vi "bf.vi"() -> ()   [LabVIEW 2012]
panel:
  in  "Standard Input":string
  out "Standard Output":string
  in  "Source Code":string
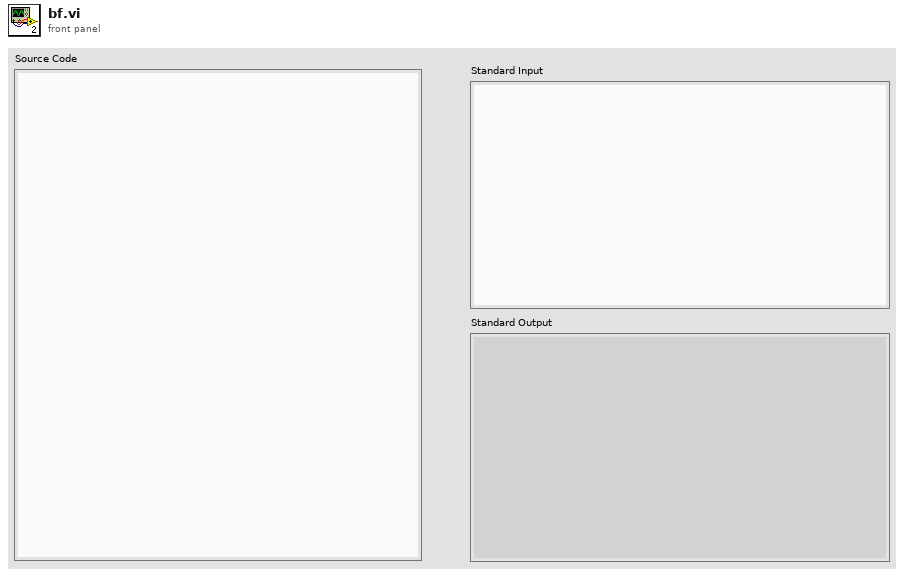
[diagram p1: front panel]
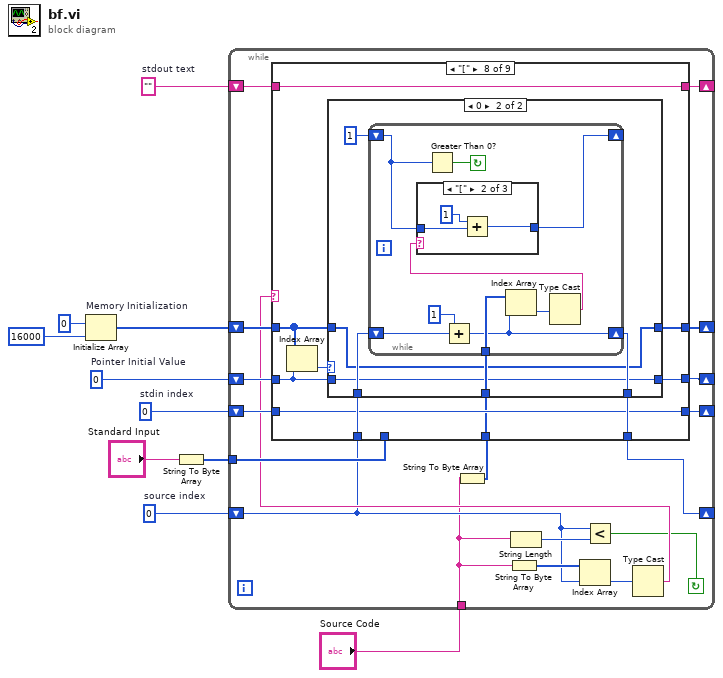
[diagram p0: block diagram]
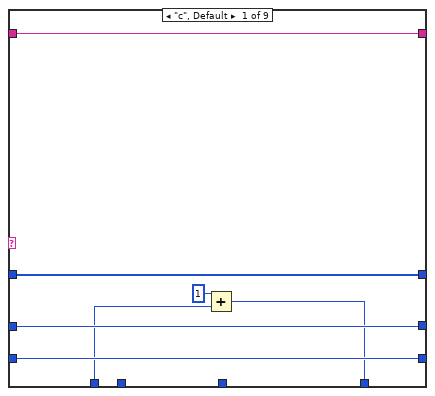
[diagram p2: hidden frame]
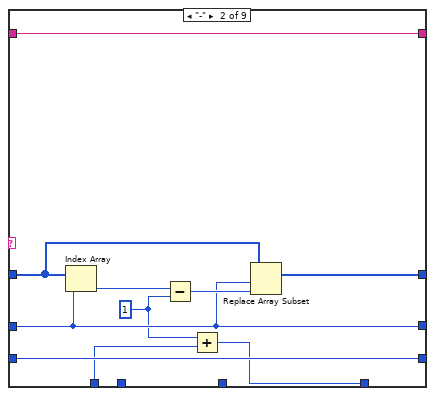
[diagram p3: hidden frame]
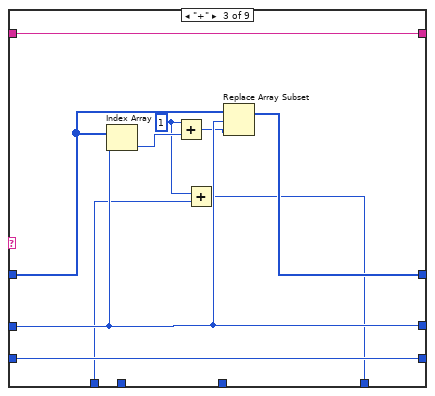
[diagram p4: hidden frame]
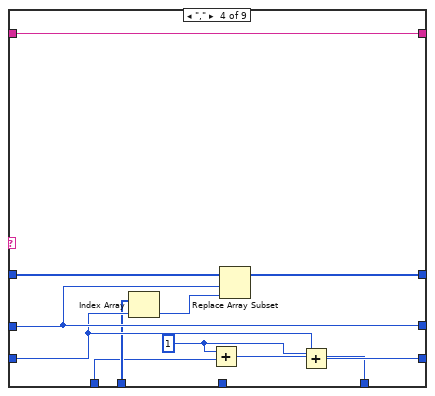
[diagram p5: hidden frame]
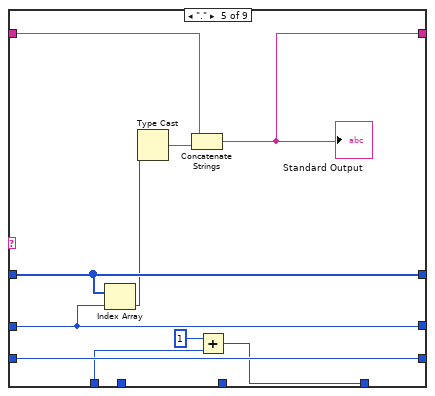
[diagram p6: hidden frame]
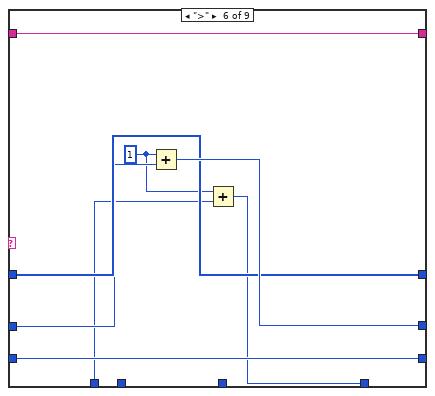
[diagram p7: hidden frame]
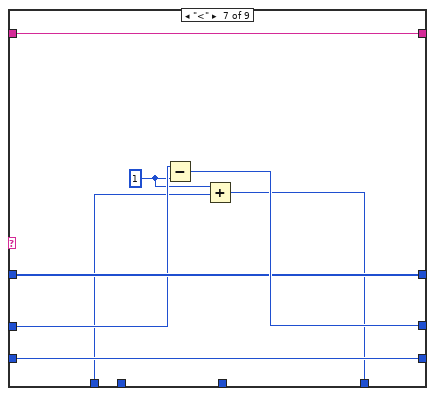
[diagram p8: hidden frame]
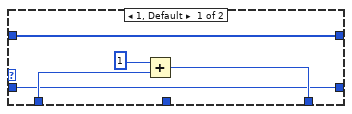
[diagram p9: hidden frame]
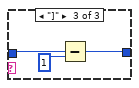
[diagram p11: hidden frame]
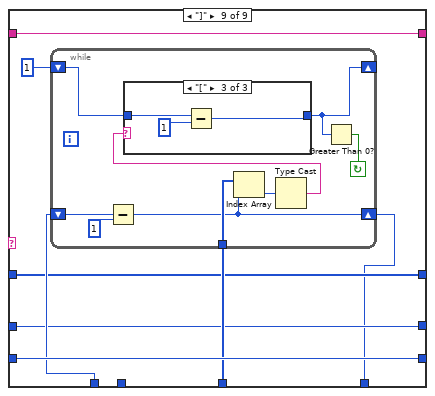
[diagram p12: hidden frame]
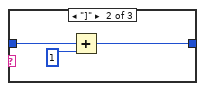
[diagram p14: hidden frame]
diagram:
  w1 = 0  # source index
  w4 = ""  # stdout text
  w5 = 0  # stdin index
  w8 = 0  # Pointer Initial Value
  n1 = Initialize Array "Memory Initialization"(u16 0, 16000) -> (w9:u16[])
  n2 = String To Byte Array(string="Standard Input") -> (unsigned byte array=w6:u8[])
  n3 = while {
    tunnel: "Source Code" -> [w12]
    shift-right: [w28] -> _
    shift-left: w8 -> [w25]
    shift-right: [w26] -> _
    shift-left: w9 -> [w27]
    tunnel: w6 -> [w22]
    shift-right: [w23] -> _
    shift-left: w5 -> [w24]
    shift-right: [w21] -> _
    shift-left: w4 -> [w20]
    shift-right: [w19] -> _
    shift-left: w1 -> [w13]
    stop <- w15 continue-if-true
    n4 = String To Byte Array(string=w12) -> (unsigned byte array=w11:u8[])
    n5 = String To Byte Array(string=w12) -> (unsigned byte array=w18:u8[])
    n6 = String Length(string=w12) -> (length=w14:i32)
    n7 = Index Array(array=w18, index=w13) -> (element=w16:u8)
    n8 = Less?(x=w13, y=w14) -> (x < y?=w15:bool)
    n9 = Type Cast(x=w16) -> (*(type *) &x=w17:string)  [unwired: 1 in]
    n10 = case shown="\"[\"" w17 {
      tunnel: [w34 w41 w52 w64 w75 w84 w92 w93 w131] -> w28
      tunnel: w27 -> [w35 w45 w53 w66 w76 w83 w91 w96 w132]
      tunnel: [w35 w44 w54 w65 w76 w83 w91 w95 w132] -> w26
      tunnel: w25 -> [w34 w41 w52 w64 w75 w82 w89 w94 w131]
      tunnel: w24 -> [w33 w40 w50 w63 w73 w81 w90 w99 w135]
      tunnel: [w33 w40 w50 w62 w73 w81 w90 w99 w135] -> w23
      tunnel: w22 -> [_ _ _ w61 _ _ _ _ _]
      tunnel: [w32 w39 w49 w59 w70 w80 w88 w97 w137] -> w21
      tunnel: w20 -> [w32 w39 w49 w59 w72 w80 w88 w97 w137]
      tunnel: w13 -> [w30 w37 w46 w57 w68 w78 w86 w101 w134]
      tunnel: [w29 w36 w47 w58 w69 w77 w85 w100 w130] -> w19
      tunnel: w11 -> [_ _ _ _ _ _ _ w98 w133]
      frame "c", Default {
        n11 = Add(x=1, y=w30) -> (x+y=w29:i32)
      }
      frame "-" {
        w38 = 1
        n12 = Index Array(array=w45, index=w41) -> (element=w43:u16)
        n13 = Subtract(x=w43, y=w38) -> (x-y=w42:i32)
        n14 = Add(x=w38, y=w37) -> (x+y=w36:i32)
        n15 = Replace Array Subset(array=w45, new element=w42, index=w41) -> (w44:u16[])
      }
      frame "+" {
        w48 = 1
        n16 = Index Array(array=w53, index=w52) -> (element=w55:u16)
        n17 = Add(x=w48, y=w55) -> (x+y=w51:i32)
        n18 = Add(x=w48, y=w46) -> (x+y=w47:i32)
        n19 = Replace Array Subset(array=w53, new element=w51, index=w52) -> (w54:u16[])
      }
      frame "," {
        w56 = 1
        n20 = Index Array(array=w61, index=w63) -> (element=w60:u8)
        n21 = Add(x=w56, y=w57) -> (x+y=w58:i32)
        n22 = Replace Array Subset(array=w66, new element=w60, index=w64) -> (w65:u16[])
        n23 = Add(x=w56, y=w63) -> (x+y=w62:i32)
      }
      frame "." {
        n24 = Index Array(array=w76, index=w75) -> (element=w74:u16)
        n25 = Type Cast(x=w74) -> (*(type *) &x=w71:string)  [unwired: 1 in]
        n26 = Concatenate Strings(w72, w71) -> (w70:string)
        "Standard Output" <- w70
        n27 = Add(x=1, y=w68) -> (x+y=w69:i32)
      }
      frame ">" {
        w79 = 1
        n28 = Add(x=w79, y=w82) -> (x+y=w84:i32)
        n29 = Add(x=w79, y=w78) -> (x+y=w77:i32)
      }
      frame "<" {
        w87 = 1
        n30 = Subtract(x=w89, y=w87) -> (x-y=w92:i32)
        n31 = Add(x=w87, y=w86) -> (x+y=w85:i32)
      }
      frame "[" {
        n32 = Index Array(array=w96, index=w94) -> (element=w102:u16)
        n33 = case shown="0" w102 {
          tunnel: w101 -> [w105 w112]
          tunnel: [w107 w111] -> w100
          tunnel: w98 -> [_ w110]
          tunnel: w96 -> [w104 w108]
          tunnel: [w104 w108] -> w95
          tunnel: w94 -> [w103 w109]
          tunnel: [w103 w109] -> w93
          frame 1, Default {
            n34 = Add(x=1, y=w105) -> (x+y=w107:i32)
          }
          frame 0 {
            n35 = while {
              shift-right: [w115] -> _
              shift-left: 1 -> [w114]
              tunnel: w110 -> [w119]
              shift-right: [w118] -> w111
              shift-left: w112 -> [w121]
              stop <- w122 continue-if-true
              n36 = Greater Than 0?(x=w114) -> (x > 0?=w122:bool)
              n37 = Add(x=1, y=w121) -> (x+y=w118:i32)
              n38 = Index Array(array=w119, index=w118) -> (element=w117:u8)
              n39 = Type Cast(x=w117) -> (*(type *) &x=w116:string)  [unwired: 1 in]
              n40 = case shown="\"[\"" w116 {
                tunnel: [w123 w124 w127] -> w115
                tunnel: w114 -> [w123 w125 w128]
                frame "0", Default {
                }
                frame "[" {
                  n41 = Add(x=1, y=w125) -> (x+y=w124:i32)
                }
                frame "]" {
                  n42 = Subtract(x=w128, y=1) -> (x-y=w127:i32)
                }
              }
            }
          }
        }
      }
      frame "]" {
        n43 = while {
          shift-right: [w142] -> w130
          shift-left: w134 -> [w145]
          tunnel: w133 -> [w143]
          shift-right: [w138] -> _
          shift-left: 1 -> [w139]
          stop <- w146 continue-if-true
          n44 = Subtract(x=w145, y=1) -> (x-y=w142:i32)
          n45 = Index Array(array=w143, index=w142) -> (element=w141:u8)
          n46 = Type Cast(x=w141) -> (*(type *) &x=w140:string)  [unwired: 1 in]
          n47 = case shown="\"[\"" w140 {
            tunnel: w139 -> [w147 w150 w152]
            tunnel: [w147 w148 w151] -> w138
            frame "1", Default {
            }
            frame "]" {
              n48 = Add(x=w150, y=1) -> (x+y=w148:i32)
            }
            frame "[" {
              n49 = Subtract(x=w152, y=1) -> (x-y=w151:i32)
            }
          }
          n50 = Greater Than 0?(x=w138) -> (x > 0?=w146:bool)
        }
      }
    }
  }
